vi "LinearFilter_MovingAvg_Execute.vi"(9 "Samples":i32=3 min=1, 10 "Enable":bool=TRUE, 11 "Input":dbl format="%13.5p") -> (1 "Output":dbl format="%13.5p")   [LabVIEW 2019, in "Trajectory_Library.lvlib"]
doc: "This is a LabVIEW \"convience\" function that combines the various subVI for a linear filter into a single subVI. This subVI creates and executes the linear filter. The filter can be dynamically enabled and disabled. When the filter is disabled, the input is transfered directly to the output. Bumpless transfer is provided when enabling the filter. Bumpless transfer is NOT provided when disabling the filter. The output value jumps directly to the current input value. The filter type and filter constants can also be changed dynamically. When the filter contstants are changed, the output may jump to the current input value when the internal buffers are reset to the current input value.\n\nInputs:\n - FilterType - An enumerated value used to select the type of filter to be cofigured. The possible values are:\n - Moving Average - Specify the \"sample\" input.\n - Low pass 1st order Butterworth filter\n - Low pass 2nd order Butterworth filter\n - High pass 1st order Butterworth filter\n - High pass 2nd order Butterworth filter\n - Input - Input value to be filtered (Required) \n - Enable - Boolean indicating filtering should be performed (Default = True)\n - TimeConstant - Filtering time constant seconds. Used for all types except Moving \n Average (Default = 0.020) \n - SamplePeriod - Execution period seconds. Used for all types except Moving Average. \n (Default = 0.020)\n - Samples - Number of samples for the moving average filter. (Default = 3)\n\nOutputs:\n - OutLinearFilter - Current value of the LinearFilter data structure.\n - Output - Current output value."
uses:
  Trajectory_Library.lvlib
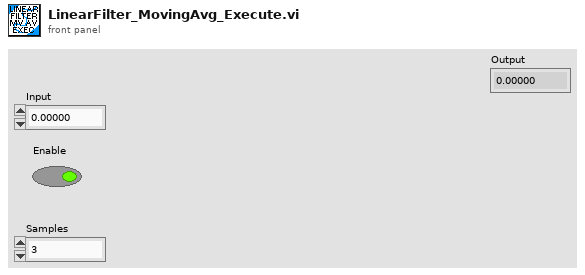
[diagram p1: front panel]
types:
  T1 = typedef "Trajectory_Library.lvlib/LINEAR_FILTER.ctl" = cluster{"InputGains":dbl[], "OutputGains":dbl[], "Inputs":dbl[], "Outputs":dbl[], "InGainCount":i32, "OutGainCount":i32}
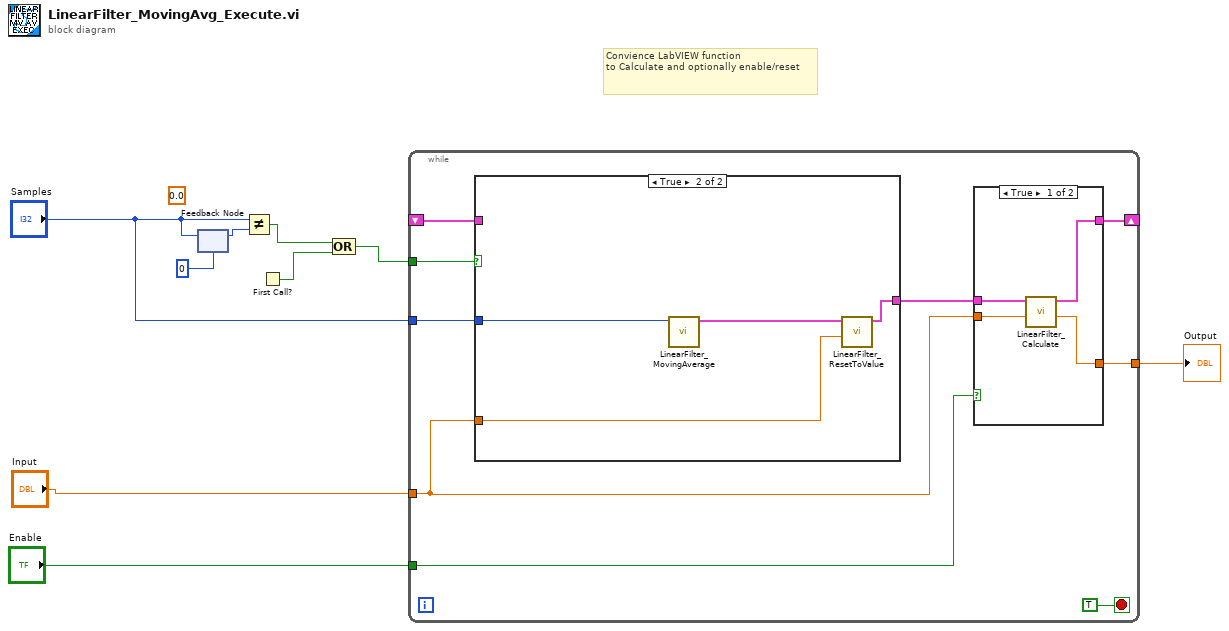
[diagram p0: block diagram]
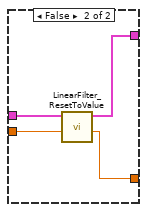
[diagram p2: hidden frame]
diagram:
  (unwired) 0.0 ("SamplePeriod")
  # "Convience LabVIEW function\nto Calculate and optionally enable/reset"
  n1 = feedback #1(0 ("Samples")) -> (w3:i32)
  n2 = feedback-in #1("Samples") -> ()
  n3 = Not Equal?(x="Samples", y=w3) -> (x != y?=w6:bool)
  n4 = First Call?() -> (First Call?: T/F=w5:bool)
  n5 = Compound Arithmetic op=OR(w6, w5) -> (w2:bool)
  n6 = while {
    tunnel: "Enable" -> [w18]
    tunnel: "Samples" -> [w14]
    tunnel: w2 -> [w12]
    tunnel: "Input" -> [w16]
    tunnel: [w17] -> w8
    shift-right: [w13] -> _
    shift-left: _ -> [w10]
    stop <- TRUE stop-if-true
    n7 = case shown="True" w12 {
      tunnel: w14 -> [_ w29]
      tunnel: w16 -> [_ w28]
      tunnel: [w26 w27] -> w15
      tunnel: w10 -> [w26 _]
      frame False {
      }
      frame True {
        n8 = call "LinearFilter_MovingAverage.vi"("Samples"=w29) -> ("LINEAR_FILTER"=w30:T1)  [unwired: 9 in, 1 out]
        n9 = call "LinearFilter_ResetToValue.vi"("InputValue"=w28, "In LINEAR_FILTER"=w30) -> ("Out LINEAR_FILTER"=w27:T1)  [unwired: 9 in]
      }
    }
    n10 = case shown="True" w18 {
      tunnel: w15 -> [w22 w25]
      tunnel: [w21 w24] -> w13
      tunnel: w16 -> [w20 w23]
      tunnel: [w19 w23] -> w17
      frame True {
        n11 = call "LinearFilter_Calculate.vi"("Input"=w20, "In LINEAR_FILTER"=w22) -> ("Output"=w19:dbl, "Out LINEAR_FILTER"=w21:T1)  [unwired: 8 in]
      }
      frame False {
        n12 = call "LinearFilter_ResetToValue.vi"("InputValue"=w23, "In LINEAR_FILTER"=w25) -> ("Out LINEAR_FILTER"=w24:T1)  [unwired: 9 in]
      }
    }
  }
  "Output" <- w8
